vi "Gas Rack AI Read.vi"(10 "Channel to Cal":T1) -> (0 "Lost Connection":bool, 2 "Available?":bool, 3 "Data":dbl format="%0.2f")   [LabVIEW 2019]
uses:
  Type Defs/Gas Rack Channel Type Def (RIO).ctl
  Type Defs/TCP Data Stream Mode (PC).ctl
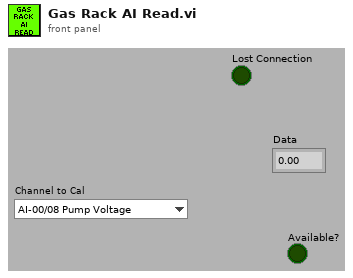
[diagram p1: front panel]
types:
  T1 = typedef "Gas Rack Channel Type Def (RIO).ctl" = enum16{"AI-00/08 Pump Voltage", "AI-01/09 Pump Current", "AI-02/10 Pressure", "AI-03/11 Flow", "AI-04/12 Controller Voltage", "AI-07/15 Controller Current", "AI-06/14 Temperature", "AI-05/13 Spare"}
  T2 = typedef "TCP Data Stream Mode (PC).ctl" = enum16{"Init", "Read Data", "Close"}
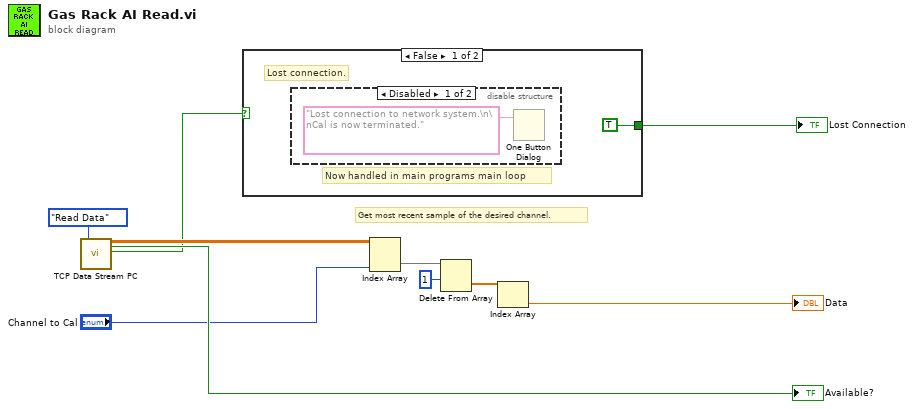
[diagram p0: block diagram]
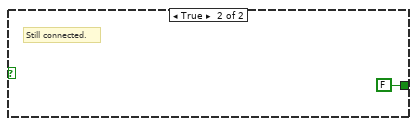
[diagram p3: hidden frame]
diagram:
  # "Get most recent sample of the desired channel."
  n1 = call "TCP Data Stream PC.vi"("Mode"=TCP_Data_Stream_Mode_(PC)."Read Data") -> ("Data OUT"=w3:dbl[][], "New Data?"=→"Available?":bool, "Connected?"=w2:bool)  [unwired: 15 in, 1 out]
  n2 = case shown="False" w2 {
    tunnel: [TRUE FALSE] -> w8
    frame False {
      # "Now handled in main programs main loop"
      # "Lost connection."
      n3 = disable-structure shown="Disabled" {
        frame Disabled {
          n4 = One Button Dialog(message="Lost connection to network system.\n\nCal is now terminated.") -> ()  [unwired: 1 in, 1 out]
        }
        frame Enabled {
        }
      }
    }
    frame True {
      # "Still connected."
    }
  }
  "Lost Connection" <- w8
  n5 = Index Array(array=w3, index (col)="Channel to Cal") -> (element=w7:dbl[])  [unwired: 1 in]
  n6 = Delete From Array(array=w7, length=1) -> (deleted portion=w5:dbl[])  [unwired: 1 in, 1 out]
  n7 = Index Array(array=w5) -> (element=→"Data":dbl)  [unwired: 1 in]
